vi "DistToObst.vi"(1 "error in (no error)":errorcluster, 2 "UTM Location":T1 {"North" format="%#_10f"; "East" format="%#_8f"}, 3 "Obstacle.lvclass":refnum<class "Obstacle.lvclass">) -> (0 "min value":dbl)   [LabVIEW 2012, in "Obstacle.lvclass"]
doc: "Takes in Obstacle and a UTM location and returns the distance to the closest point in the object.\nPerpetrator: Michael Bocamazo"
uses:
  Obstacle.lvclass
  Data/TypeDefs/UTM Location.ctl
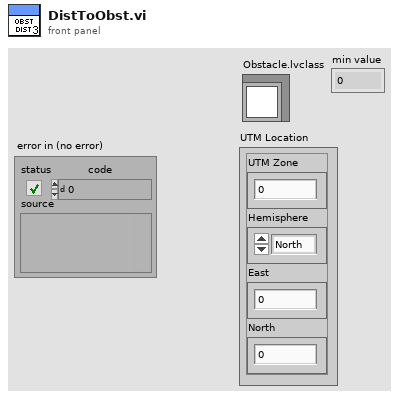
[diagram p1: front panel]
types:
  T1 = typedef "UTM Location.ctl" = cluster{"UTM Zone":dbl, "Hemisphere":enum16{"North", "South"}, "East":dbl, "North":dbl}
  T2 = cluster{"UTM Location 2":T1, "UTM Location":T1}[]
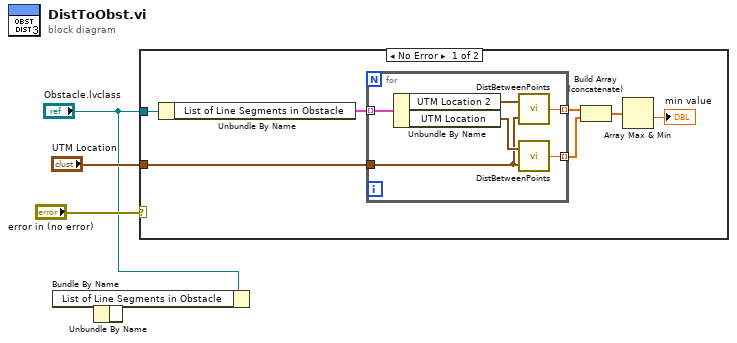
[diagram p0: block diagram]
diagram:
  n1 = Bundle By Name(cluster="Obstacle.lvclass") -> ()  [unwired: 1 in, 1 out]
  n2 = Unbundle By Name() -> ()  [unwired: 1 in, 1 out]
  n3 = case shown="No Error" "error in (no error)" {
    tunnel: "Obstacle.lvclass" -> [w10 _]
    tunnel: "UTM Location" -> [w8 _]
    frame No Error {
      n4 = Unbundle By Name(w10) -> ("List of Line Segments in Obstacle"=w9:T2)
      n5 = for {
        tunnel: w9 -> [w16] mode=indexing
        tunnel: w8 -> [w13]
        tunnel: [w12] -> w6 mode=indexing
        tunnel: [w11] -> w5 mode=indexing
        n6 = Unbundle By Name(w16) -> ("UTM Location 2"=w15:T1, "UTM Location"=w14:T1)
        n7 = call "DistBetweenPoints.vi"("UTM Location 2"=w13, "UTM Location"=w15) -> ("Numeric"=w12:dbl)
        n8 = call "DistBetweenPoints.vi"("UTM Location 2"=w13, "UTM Location"=w14) -> ("Numeric"=w11:dbl)
      }
      n9 = Build Array (concatenate)(w6, w5) -> (w4:dbl[])
      n10 = Array Max & Min(array=w4) -> (min value=→"min value":dbl)  [unwired: 3 out]
    }
    frame Error {
    }
  }
